vi "Module Init.vi"(8 "error in (no error)":errorcluster, 11 "DAQmxAI in":refnum<class "DAQmxAI.lvclass">) -> (0 "error out":errorcluster, 3 "DAQmxAI out":refnum<class "DAQmxAI.lvclass">)   [LabVIEW 2023, in "VolatusDAQ.lvlib" / "DAQmxAI.lvclass"]
uses:
  DAQmxAI.lvclass
  DAQmxAI.lvclass/DAQmxAI.ctl
  Volatus/Module/Module.lvclass/Module.ctl
  Volatus/MessageQ/MessageQ.lvclass/MessageQ.ctl
  Volatus/Module/Self Q.vi
  Volatus/MessageQ/Send.vi
  Volatus/Module/Module.lvclass
  VolatusData/Data Processor Module/Data Processor Module.lvclass
  VolatusDAQ.lvlib
  C:/dev/volatus/mts-volatus-super/libs/lv-volatus/Volatus/Module/Module.lvclass
  C:/dev/volatus/mts-volatus-super/libs/lv-volatus/VolatusDAQ/DAQmxAI/DAQmxAI.lvclass
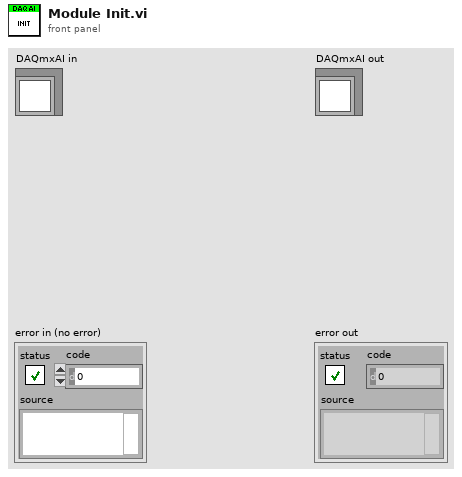
[diagram p1: front panel]
types:
  T1 = typedef "VolatusDAQConfig.lvlib/Sampling Config.ctl" = cluster{"Rate":dbl, "Chunk Size":i32}
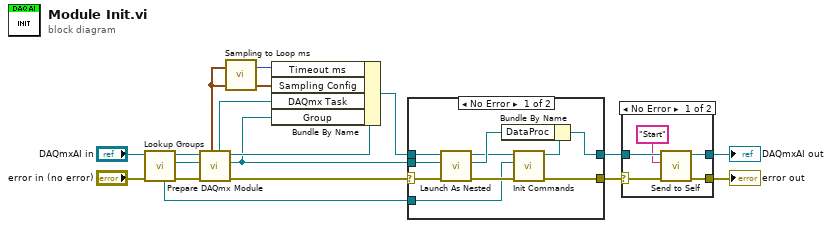
[diagram p0: block diagram]
diagram:
  n1 = call "Lookup Groups.vi"("error in (no error)"="error in (no error)", "DAQmxAI in"="DAQmxAI in") -> ("error out"=w5:errorcluster, "Channels"=w2:refnum<class "Group Config.lvclass">, "DAQmxAI out"=w3:refnum<class "DAQmxAI.lvclass">, "Commands"=w1:refnum<class "Group Config.lvclass">)  [unwired: 6 in]
  n2 = call "Prepare DAQmx Module.vi"("error in (no error)"=w5, "Group Config (Lookup)"=w2, "Module in"=w3) -> ("error out"=w10:errorcluster, "Group"=w8:refnum<class "Group DBL.lvclass">, "Module out"=w12:refnum<class "DAQmxAI.lvclass">, "DAQmx Task"=w9:refnum<k21>, "Sampling Config"=w7:T1)  [unwired: 3 in, 1 out]
  n3 = call "Sampling to Loop ms.vi"("Sampling Config"=w7) -> ("Loop Timeout ms"=w6:i32)  [unwired: 6 in]
  n4 = Bundle By Name(cluster=w12, "Timeout ms"=w6, "Sampling Config"=w7, "DAQmx Task"=w9, "Group"=w8) -> (w11:refnum<class "DAQmxAI.lvclass">)
  n5 = case shown="No Error" w10 {
    selector: w10 -> [w26 w28]
    tunnel: w11 -> [w27 w29]
    tunnel: [w21 w28] -> w17
    tunnel: [w24 w29] -> w15
    tunnel: w8 -> [w22 _]
    tunnel: w1 -> [w18 _]
    frame No Error {
      n6 = call "Launch As Nested.vi"("error in (no error)"=w26, "Group"=w22, "Parent in"=w27) -> ("error out"=w23:errorcluster, "MessageQ"=w25:refnum<class "MessageQ.lvclass">, "Parent out"=w20:refnum<class "DAQmxAI.lvclass">)  [unwired: 6 in]
      n7 = call "Init Commands.vi"("error in (no error)"=w23, "Commands"=w18, "DAQmxAI in"=w20) -> ("error out"=w21:errorcluster, "DAQmxAI out"=w19:refnum<class "DAQmxAI.lvclass">)  [unwired: 7 in]
      n8 = Bundle By Name(cluster=w19, "DataProc"=w25) -> (w24:refnum<class "DAQmxAI.lvclass">)
    }
    frame Error {
    }
  }
  n9 = case shown="No Error" w17 {
    selector: w17 -> [w34 w36]
    tunnel: [w33 w36] -> w16
    tunnel: w15 -> [w32 w35]
    tunnel: [w31 w35] -> w14
    frame No Error {
      n10 = call "Send to Self.vi"("error in (no error)"=w34, "Message ID"="Start", "Module in"=w32) -> ("error out"=w33:errorcluster, "Module out"=w31:refnum<class "DAQmxAI.lvclass">)  [unwired: 7 in]
    }
    frame Error {
    }
  }
  "error out" <- w16
  "DAQmxAI out" <- w14
